vi "Periodic Tasks.vi"(8 "error in":errorcluster) -> ()   [LabVIEW 2020]
doc: "This VI runs in parallel to other tasks. It can contain as many user-defined periodic loops as you need. These can carry out PID or other sorts of timed response."
uses:
  <vilib>/Rock Robotics/WPI/ThirdParty/Phoenix-LabVIEW/Motor Controller/Controls/CTRE_Phoenix_MotorControl_ControlMode.ctl
  <vilib>/Rock Robotics/WPI/Utilities/WPI_GetSetVariantRefNum.vi
  <vilib>/Rock Robotics/WPI/ThirdParty/Phoenix-LabVIEW/Motor Controller/Get/CTRE_Phoenix_MotorController_GetSelectedSensorData.vi
  Robot Global Data.vi
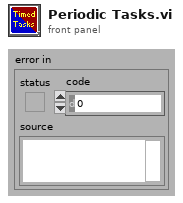
[diagram p1: front panel]
types:
  T1 = typedef "WPI_JoystickDevRef.ctl" = cluster{"Device":T2}
  T2 = typedef "WPI_JoystickDeviceEnum.ctl" = enum16{"USB 0", "USB 1", "USB 2", "USB 3", "USB 4", "USB 5"}
  T3 = typedef "WPI_RobotDriveDevRef.ctl" = cluster{"DevStatus":errorcluster, "Motors[]":T4[], "Square Inputs":bool, "Max Output":dbl}
  T4 = typedef "WPI_MotorControlDeviceRef.ctl" = cluster{"DeviceStatus":errorcluster, "Type":T5, "PWM":cluster{"PWM Channel":T6, "DeadBand":T7}, "CAN":cluster{"Device Number":u8, "SetOutput VI Ref":variant, "GetOutput VI Ref":variant, "Enable VI Ref":variant, "Disable VI Ref":variant, "Data":variant}, "Invert":bool, "DIO PWM":cluster{"PWM \"Enable\" Channel":T6, "DIOChannel":T8, "PWM Rate":dbl}}
  T5 = typedef "WPI_MotorControlType.ctl" = enum16{"PWM", "CAN", "DIO PWM"}
  T6 = typedef "FPGA_DIOPWMChannel.ctl" = enum8{"PWM 0", "PWM 1", "PWM 2", "PWM 3", "PWM 4", "PWM 5", "PWM 6", "PWM 7", "PWM 8", "PWM 9", "PWM MXP 0", "PWM MXP 1", "PWM MXP 2", "PWM MXP 3", "PWM MXP 4", "PWM MXP 5", "PWM MXP 6", "PWM MXP 7", "PWM MXP 8", "PWM MXP 9", "Invalid"}
  T7 = typedef "WPI_PWMDeadband.ctl" = cluster{"Name":string, "maxPositivePwm":i32, "minPositivePwm":i32, "centerPwm":i32, "maxNegativePwm":i32, "minNegativePwm":i32, "angularRange":u16}
  T8 = typedef "FPGA_DIOChannel.ctl" = enum8{"DIO 0", "DIO 1", "DIO 2", "DIO 3", "DIO 4", "DIO 5", "DIO 6", "DIO 7", "DIO 8", "DIO 9", "DIO MXP 0", "DIO MXP 1", "DIO MXP 2", "DIO MXP 3", "DIO MXP 4", "DIO MXP 5", "DIO MXP 6", "DIO MXP 7", "DIO MXP 8", "DIO MXP 9", "DIO MXP 10", "DIO MXP 11", "DIO MXP 12", "DIO MXP 13", "DIO MXP 14", "DIO MXP 15", "SPI Port CS1", "SPI Port CS2", "SPI Port CS3", "SPI Port MISO", "SPI Port MOSI", "Invalid"}
  T9 = cluster{"JoystickDevRef":T1, "RobotDriveDevRef":T3}
  T10 = typedef "CTRE_Phoenix_MotorControl_ControlMode.ctl" = u16
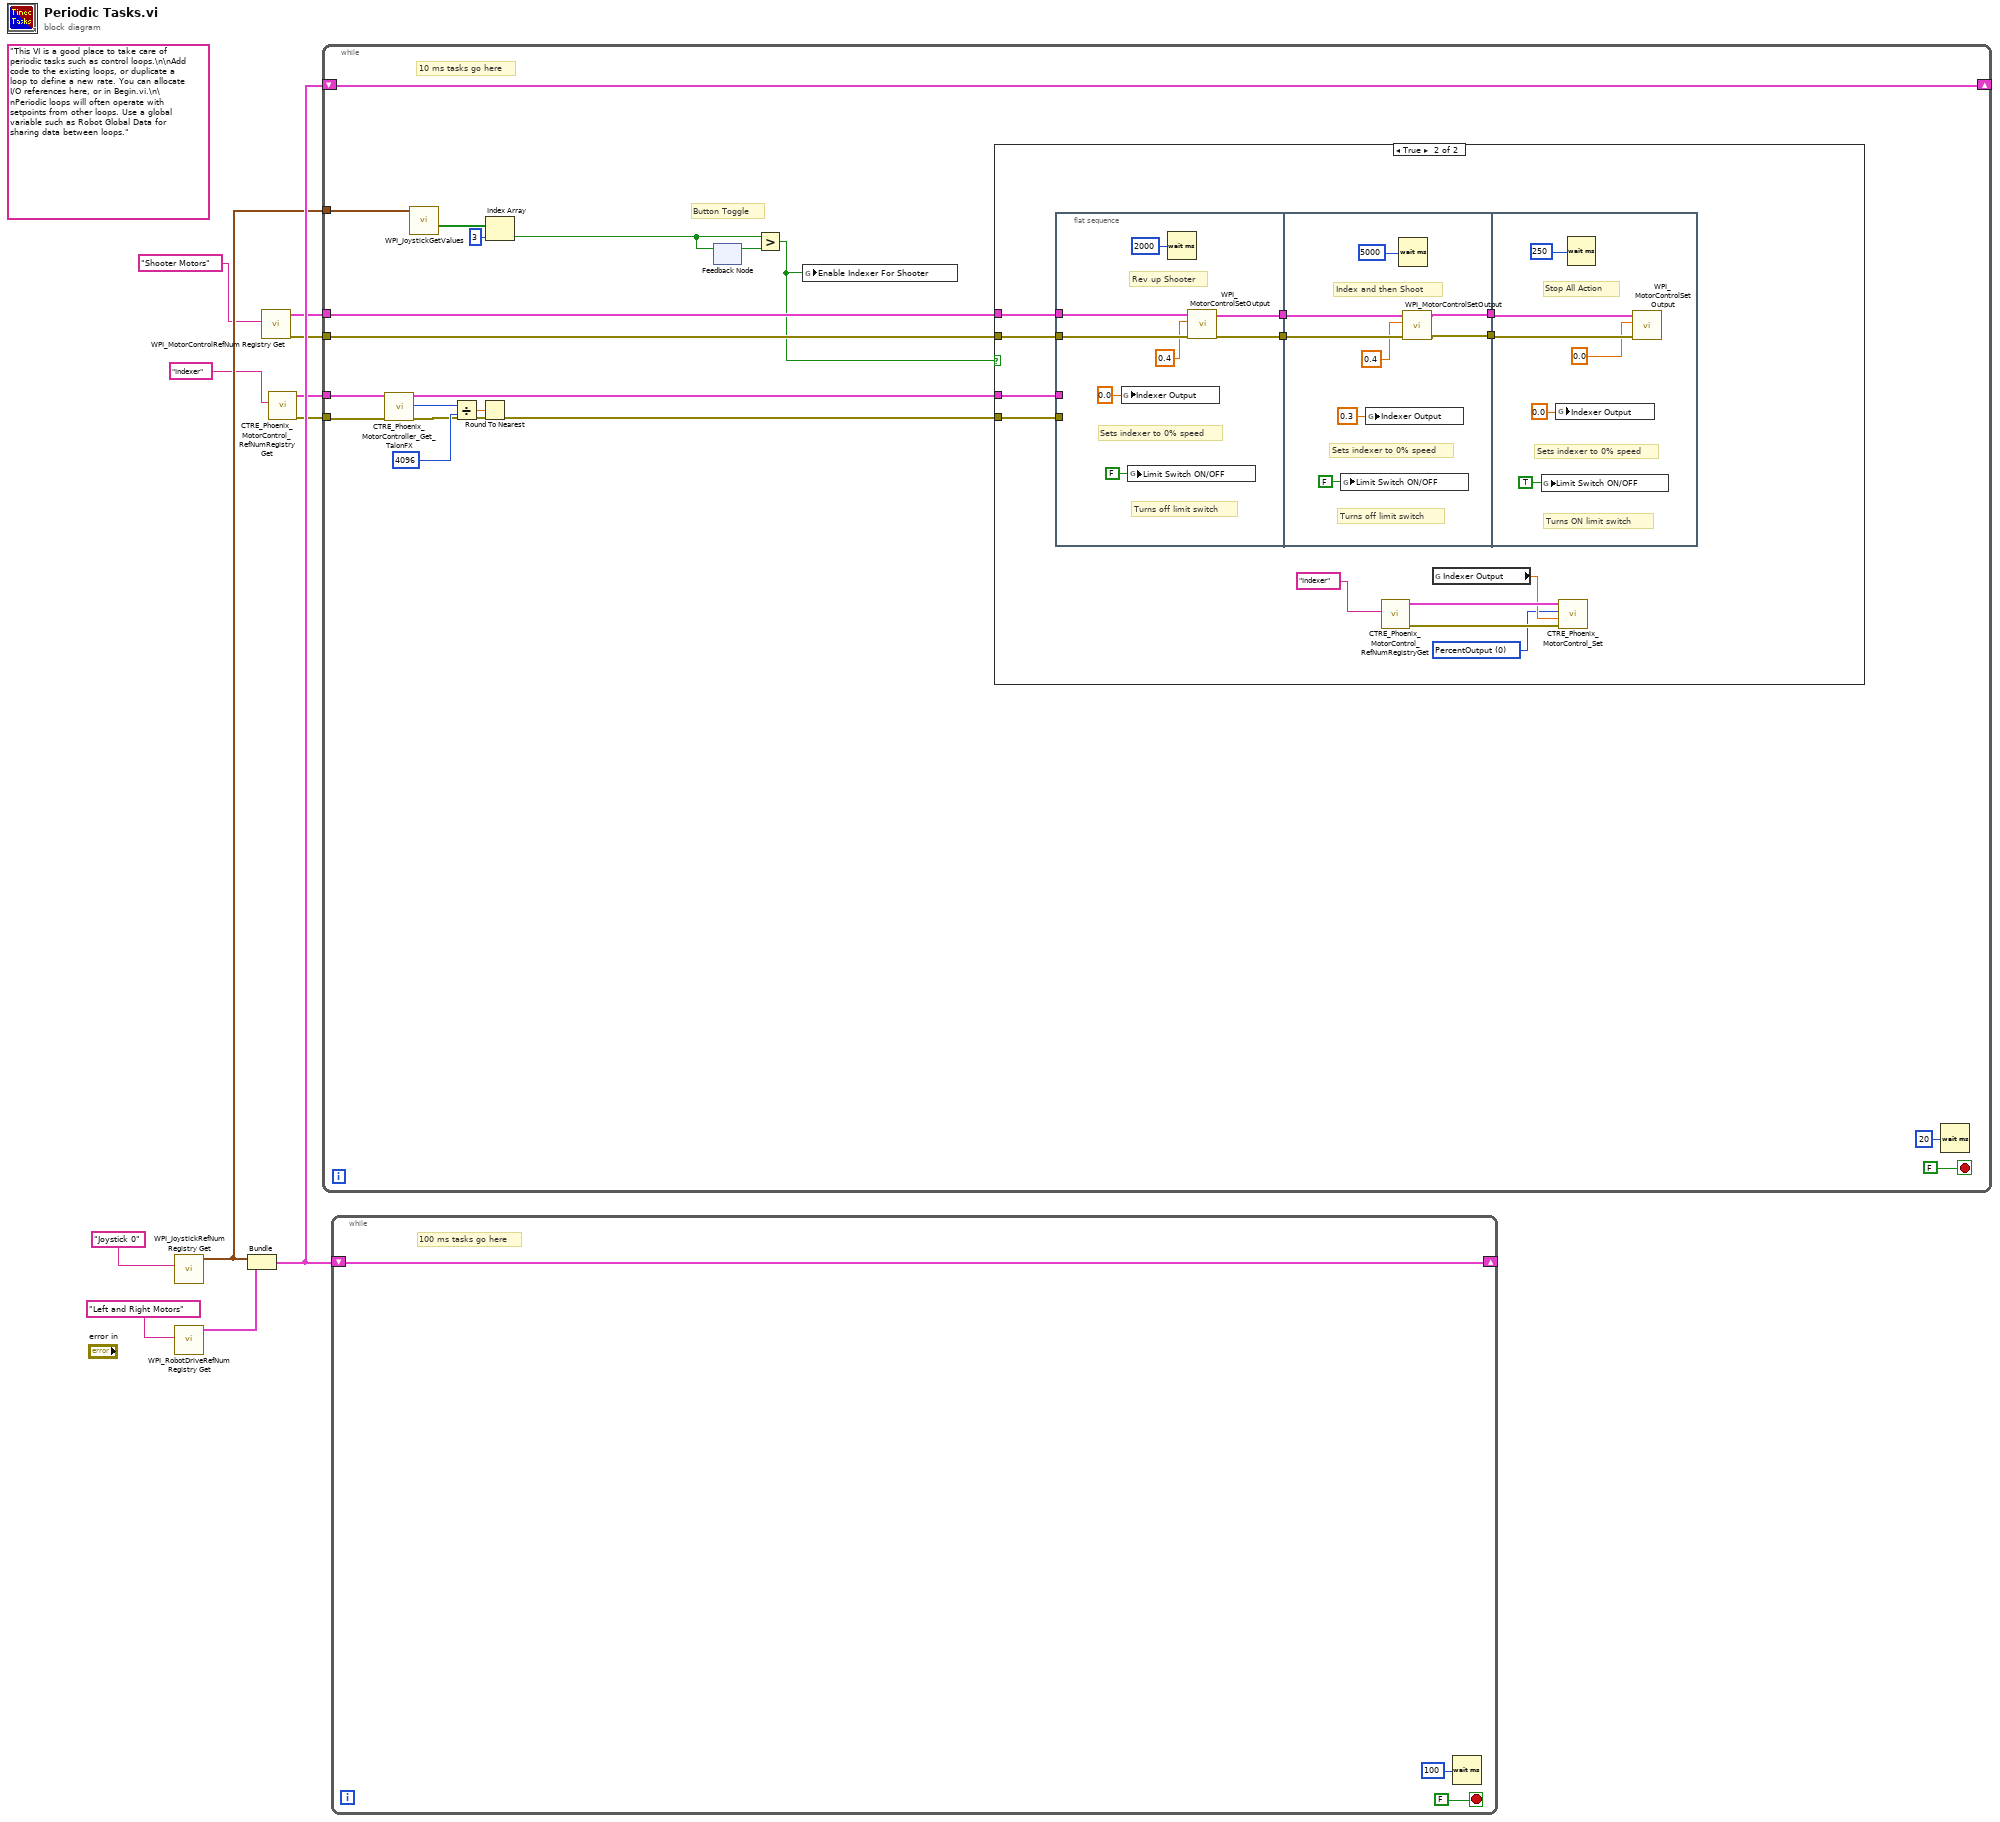
[diagram p0: block diagram]
diagram:
  (unwired) "This VI is a good place to take care of periodic tasks such as control loops.\n\nAdd code to the existing loops, or duplicate a loop to define a new rate. You can allocate I/O references here, or in Begin.vi.\n\nPeriodic loops will often operate with setpoints from other loops. Use a global variable such as Robot Global Data for sharing data between loops."
  n1 = call <vilib>:"WPI_JoystickRefNum Registry Get.vi"("refnum name"="Joystick 0") -> ("JoystickDevRef"=w7:T1)  [unwired: 1 in, 9 out]
  n2 = call <vilib>:"WPI_RobotDriveRefNum Registry Get.vi"("refnum name"="Left and Right Motors") -> ("RobotDriveDevRef"=w9:T3)  [unwired: 1 in, 9 out]
  n3 = Bundle("JoystickDevRef"=w7, "RobotDriveDevRef"=w9) -> (w8:T9)  [unwired: 1 out]
  n4 = call <vilib>:"WPI_MotorControlRefNum Registry Get.vi"("refnum name"="Shooter Motors") -> ("error out"=w3:errorcluster, "MotorControlDevRef"=w4:T4)  [unwired: 9 in]
  n5 = call <vilib>:"CTRE_Phoenix_MotorControl_RefNumRegistryGet.vi"("refnum name"="Indexer") -> ("error out"=w1:errorcluster, "PhoenixMotorControlDevRef"=w2:T4)  [unwired: 9 in]
  n6 = while {
    shift-right: [w27] -> _
    shift-left: w8 -> [w27]
    tunnel: w7 -> [w24]
    tunnel: w4 -> [w17]
    tunnel: w3 -> [w16]
    tunnel: w2 -> [w22]
    tunnel: w1 -> [w21]
    stop <- FALSE stop-if-true
    # "Button Toggle"
    # "10 ms tasks go here"
    n7 = call-poly <vilib>:"CTRE_Phoenix_MotorController_Get_TalonFX.vi"("PhoenixMotorControlDevRef"=w22, "error in"=w21) -> ("PhoenixMotorControlDevRef"=w15:T4, "Velocity (Raw Sensor Units per 100 ms)"=w20:i32, "error out"=w14:errorcluster)  [unwired: 10 in, 1 out]
    n8 = call <vilib>:"WPI_JoystickGetValues.vi"("JoystickDevRef"=w24) -> ("Buttons"=w26:bool[])  [unwired: 6 in, 4 out]
    n9 = Divide(x=w20, y=4096) -> (x/y=w18:dbl)
    n10 = Round To Nearest(number=w18) -> ()  [unwired: 1 out]
    n11 = Index Array(array=w26, index=3) -> (element=w13:bool)
    n12 = feedback-in #1(w13) -> ()
    n13 = feedback #1() -> (w23:bool)  [unwired: 1 in]
    n14 = Greater?(x=w13, y=w23) -> (0:w12:bool)
    n15 = global write "Robot Global Data.vi" "Enable Indexer For Shooter"(w12) -> ()
    n16 = case shown="True" w12 {
      tunnel: w17 -> [_ w42]
      tunnel: w16 -> [_ w41]
      tunnel: w15 -> [_ w38]
      tunnel: w14 -> [_ w35]
      frame False {
      }
      frame True {
        w30 = T10 0 items=["PercentOutput"=0, "Position"=1, "Velocity"=2, "Current"=3, "Follower"=5, "MotionProfile"=6, "MotionMagic"=7, "MotionProfileArc"=10, "Disabled"=15] ("Control Mode")
        n17 = flat-sequence {
          tunnel: [w47] -> w40
          tunnel: [w46] -> w39
          tunnel: w42 -> [w50]
          tunnel: w41 -> [w49]
          tunnel: w38 -> [_]
          tunnel: w35 -> [_]
          tunnel: w40 -> [w57]
          tunnel: w39 -> [w56]
          tunnel: [w55] -> w37
          tunnel: [w54] -> w36
          tunnel: w37 -> [w64]
          tunnel: w36 -> [w63]
          frame #0 {
            # "Sets indexer to 0% speed"
            # "Rev up Shooter"
            # "Turns off limit switch"
            n18 = global write "Robot Global Data.vi" "Indexer Output"(0.0 ("Indexer Output")) -> ()
            n19 = global write "Robot Global Data.vi" "Limit Switch ON/OFF"(FALSE ("Limit Switch ON/OFF")) -> ()
            n20 = Wait (ms)(milliseconds to wait=u32 2000) -> ()  [unwired: 1 out]
            n21 = call <vilib>:"WPI_MotorControlSetOutput.vi"("error in (no error)"=w49, "Output"=0.4, "MotorControlDevRef"=w50) -> ("error out"=w46:errorcluster, "MotorControlDevRef"=w47:T4)  [unwired: 6 in, 1 out]
          }
          frame #1 {
            # "Sets indexer to 0% speed"
            # "Turns off limit switch"
            # "Index and then Shoot"
            n22 = global write "Robot Global Data.vi" "Limit Switch ON/OFF"(FALSE ("Limit Switch ON/OFF")) -> ()
            n23 = global write "Robot Global Data.vi" "Indexer Output"(0.3 ("Indexer Output")) -> ()
            n24 = Wait (ms)(milliseconds to wait=u32 5000) -> ()  [unwired: 1 out]
            n25 = call <vilib>:"WPI_MotorControlSetOutput.vi"("error in (no error)"=w56, "Output"=0.4, "MotorControlDevRef"=w57) -> ("error out"=w54:errorcluster, "MotorControlDevRef"=w55:T4)  [unwired: 6 in, 1 out]
          }
          frame #2 {
            # "Sets indexer to 0% speed"
            # "Turns ON limit switch"
            # "Stop All Action"
            n26 = global write "Robot Global Data.vi" "Limit Switch ON/OFF"(TRUE ("Limit Switch ON/OFF")) -> ()
            n27 = global write "Robot Global Data.vi" "Indexer Output"(0.0 ("Indexer Output")) -> ()
            n28 = Wait (ms)(milliseconds to wait=u32 250) -> ()  [unwired: 1 out]
            n29 = call <vilib>:"WPI_MotorControlSetOutput.vi"("error in (no error)"=w63, "Output"=0.0, "MotorControlDevRef"=w64) -> ()  [unwired: 6 in, 3 out]
          }
        }
        n30 = call <vilib>:"CTRE_Phoenix_MotorControl_RefNumRegistryGet.vi"("refnum name"="Indexer") -> ("error out"=w32:errorcluster, "PhoenixMotorControlDevRef"=w33:T4)  [unwired: 9 in]
        n31 = global read "Robot Global Data.vi" "Indexer Output"() -> (w31:dbl)
        n32 = call <vilib>:"CTRE_Phoenix_MotorControl_Set.vi"("error in (no error)"=w32, "Output"=w31, "Control Mode"=w30, "PhoenixMotorControlDevRef"=w33) -> ()  [unwired: 6 in, 2 out]
      }
    }
    n33 = Wait (ms)(milliseconds to wait=u32 20) -> ()  [unwired: 1 out]
  }
  n34 = while {
    shift-right: [w65] -> _
    shift-left: w8 -> [w65]
    stop <- FALSE stop-if-true
    # "100 ms tasks go here"
    n35 = Wait (ms)(milliseconds to wait=u32 100) -> ()  [unwired: 1 out]
  }
